vi "Insert_Extra_Chs.vi"() -> (5 "Plug in titles":string[](array[string]), 7 "Plug in values":string[](array[string]))   [LabVIEW 2010]
uses:
  Globals/Meas_global.vi
  Plug in sub vis/Extra_info.vi
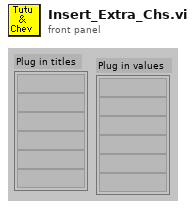
[diagram p1: front panel]
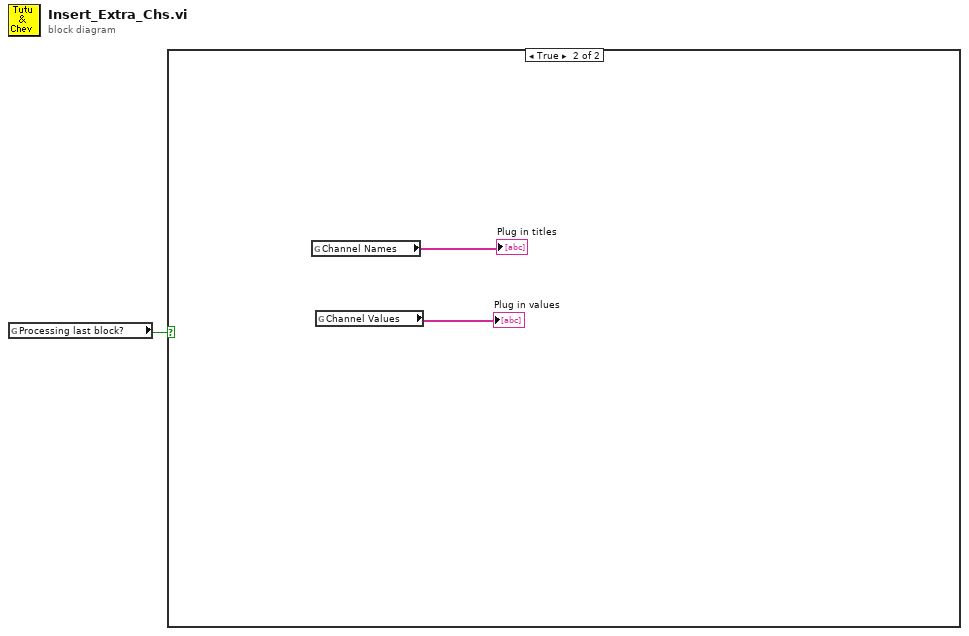
[diagram p0: block diagram]
diagram:
  n1 = global read "Meas_global.vi" "Processing last block?"() -> (w1:bool)
  n2 = case shown="True" w1 {
    frame False {
    }
    frame True {
      n3 = global read "Extra_info.vi" "Channel Names"() -> (→"Plug in titles":string[])
      n4 = global read "Extra_info.vi" "Channel Values"() -> (→"Plug in values":string[])
    }
  }
